vi "decode access token response.vi"(8 "error in (no error)":errorcluster, 9 "Response":string, 10 "Header":string, 11 "Oauth2.Salesforce in":refnum<class "Oauth2.Salesforce.lvclass">) -> (0 "error out":errorcluster, 3 "Oauth2.Salesforce":refnum<class "Oauth2.Salesforce.lvclass">)   [LabVIEW 2017, in "Oauth2.Salesforce.lvclass"]
uses:
  Oauth2.Salesforce.lvclass
  D:/GitHub/Oauth2/source/Oauth2/Oauth2.lvclass
  Oauth2/Oauth2.lvclass
  OAuthToken/OAuth2 Token Element -- enum.ctl
  OAuthToken/OAuthAccessToken.lvclass
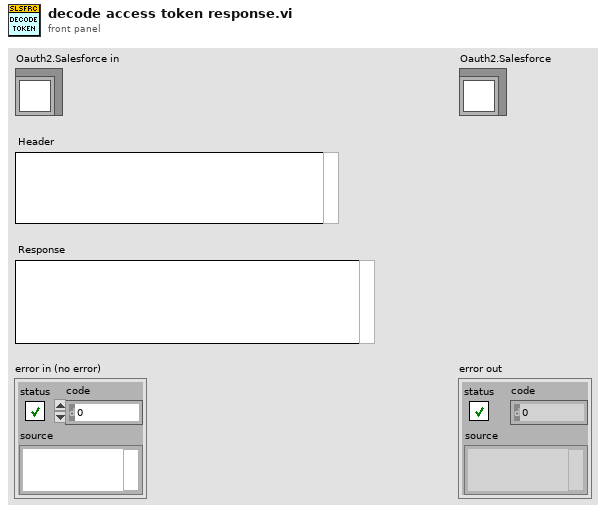
[diagram p1: front panel]
types:
  T1 = typedef "OAuthAccessToken.lvclass/OAuth2 Token Element -- enum.ctl" = enum16{"client_id", "client_secret", "response_type", "scope", "redirect_uri", "error", "error_description", "error_uri", "grant_type", "code", "access_token", "token_type", "expires_in", "username", "password", "refresh_token", "code_challenge", "code_challenge_method", "reverse_proxy_uri", "endpoint element"}
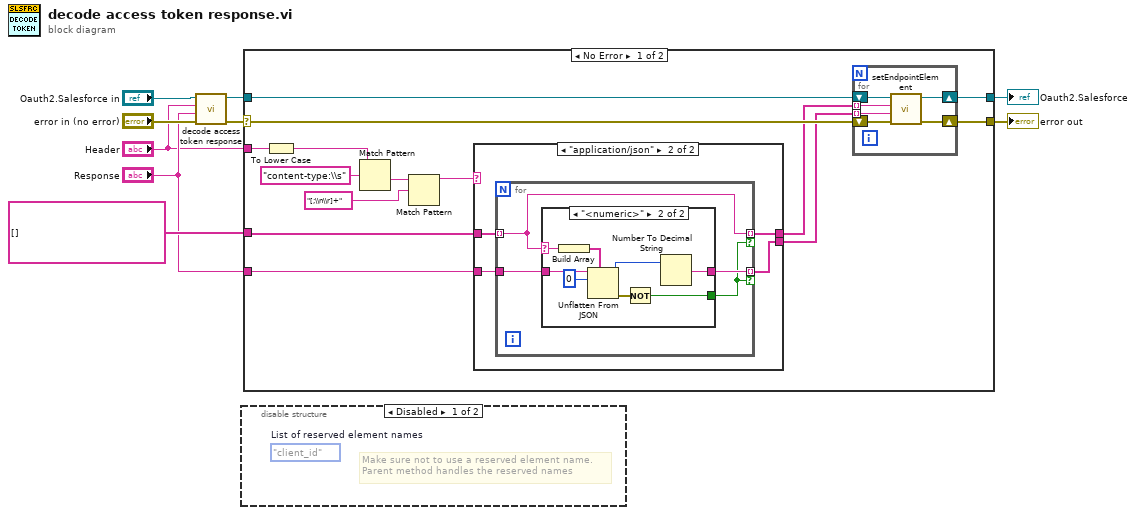
[diagram p0: block diagram]
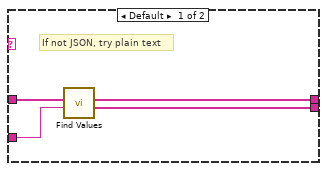
[diagram p3: hidden frame]
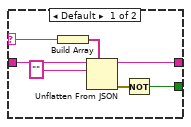
[diagram p4: hidden frame]
diagram:
  n1 = call-parent "decode access token response.vi"("error in (no error)"="error in (no error)", "Response"="Response", "Header"="Header", "Oauth2 in"="Oauth2.Salesforce in") -> ("error out"=w3:errorcluster, "Oauth2"=w4:refnum<class "Oauth2.Salesforce.lvclass">)  [unwired: 6 in]
  n2 = disable-structure shown="Disabled" {
    frame Disabled {
      (unwired) OAuth2_Token_Element_--_enum."client_id"  # List of reserved element names
      # "Make sure not to use a reserved element name.\nParent method handles the reserved names"
    }
    frame Enabled {
    }
  }
  n3 = case shown="No Error" w3 {
    selector: w3 -> [w20 w58]
    tunnel: [w21 w58] -> w1
    tunnel: [w22 w57] -> w2
    tunnel: w4 -> [w23 w57]
    tunnel: "Response" -> [w12 _]
    tunnel: "Header" -> [w19 _]
    tunnel: string[] [] -> [w13 _]
    frame No Error {
      n4 = To Lower Case(string=w19) -> (all lower case string=w15:string)
      n5 = Match Pattern(string=w15, regular expression="content-type:\\s") -> (after substring=w17:string)  [unwired: 1 in, 3 out]
      n6 = Match Pattern(string=w17, regular expression="[;\\n\\r]+") -> (before substring=w14:string)  [unwired: 1 in, 3 out]
      n7 = case shown="\"application/json\"" w14 {
        tunnel: w12 -> [w27 w31]
        tunnel: w13 -> [w24 w29]
        tunnel: [w26 w28] -> w11
        tunnel: [w25 w30] -> w10
        frame Default {
          # "If not JSON, try plain text"
          n8 = call "Find Values.vi"("Response string"=w27, "keys"=w24) -> ("values"=w25:string[], "keys dup"=w26:string[])  [unwired: 8 in]
        }
        frame "application/json" {
          n9 = for {
            tunnel: w31 -> [w35]
            tunnel: [w34] -> w30 mode=indexing if=w33
            tunnel: w29 -> [w32] mode=indexing
            tunnel: [w32] -> w28 mode=indexing if=w33
            n10 = case shown="\"<numeric>\"" w32 {
              selector: w32 -> [w36 w45]
              tunnel: w35 -> [w42 w50]
              tunnel: [w40 w43] -> w34
              tunnel: [w38 w47] -> w33
              frame Default {
                n11 = Build Array(w36) -> (w37:string[])
                n12 = Unflatten From JSON(path=w37, JSON string=w42, type and defaults="") -> (value=w40:string, error out=w39:errorcluster)  [unwired: 4 in]
                n13 = Not(x=w39) -> (.not. x?=w38:bool)
              }
              frame "<numeric>" {
                n14 = Build Array(w45) -> (w46:string[])
                n15 = Unflatten From JSON(path=w46, JSON string=w50, type and defaults=u32 0) -> (value=w44:u32, error out=w48:errorcluster)  [unwired: 4 in]
                n16 = Not(x=w48) -> (.not. x?=w47:bool)
                n17 = Number To Decimal String(number=w44) -> (decimal integer string=w43:string)  [unwired: 1 in]
              }
            }
          }
        }
      }
      n18 = for {
        shift-right: [w55] -> w22
        shift-left: w23 -> [w56]
        shift-right: [w54] -> w21
        shift-left: w20 -> [w53]
        tunnel: w11 -> [w52] mode=indexing
        tunnel: w10 -> [w51] mode=indexing
        n19 = call "setEndpointElement.vi"("error in (no error)"=w53, "Value"=w51, "Endpoint Name"=w52, "Oauth2 in"=w56) -> ("error out"=w54:errorcluster, "Oauth2 out"=w55:refnum<class "Oauth2.Salesforce.lvclass">)  [unwired: 6 in]
      }
    }
    frame Error {
    }
  }
  "error out" <- w1
  "Oauth2.Salesforce" <- w2
